vi "GetSlopeConductance3.vi"(8 "XYGraph Refnum":refnum<vi>, 10 "CapacitanceRecords":T2[](array[typedef]), 11 "Array in":dbl[][](array[numeric])) -> (1 "CleanedIV":cluster{dbl[], dbl[]}[](array[cluster]), 3 "InfoCluster":T1)   [LabVIEW 2020]
uses:
  CapacitanceRecord.ctl
  CapacitanceInfos.ctl
  <vilib>/Analysis/6fits.llb/Curve Fitting Criteria.ctl
  <vilib>/Analysis/NI_AALPro.lvlib
panel:
  out "error out":errorcluster
  out "XY Graph 2":cluster{dbl[], dbl[]}[](graph)
  out "XY Graph":cluster{dbl[], dbl[]}[](graph)
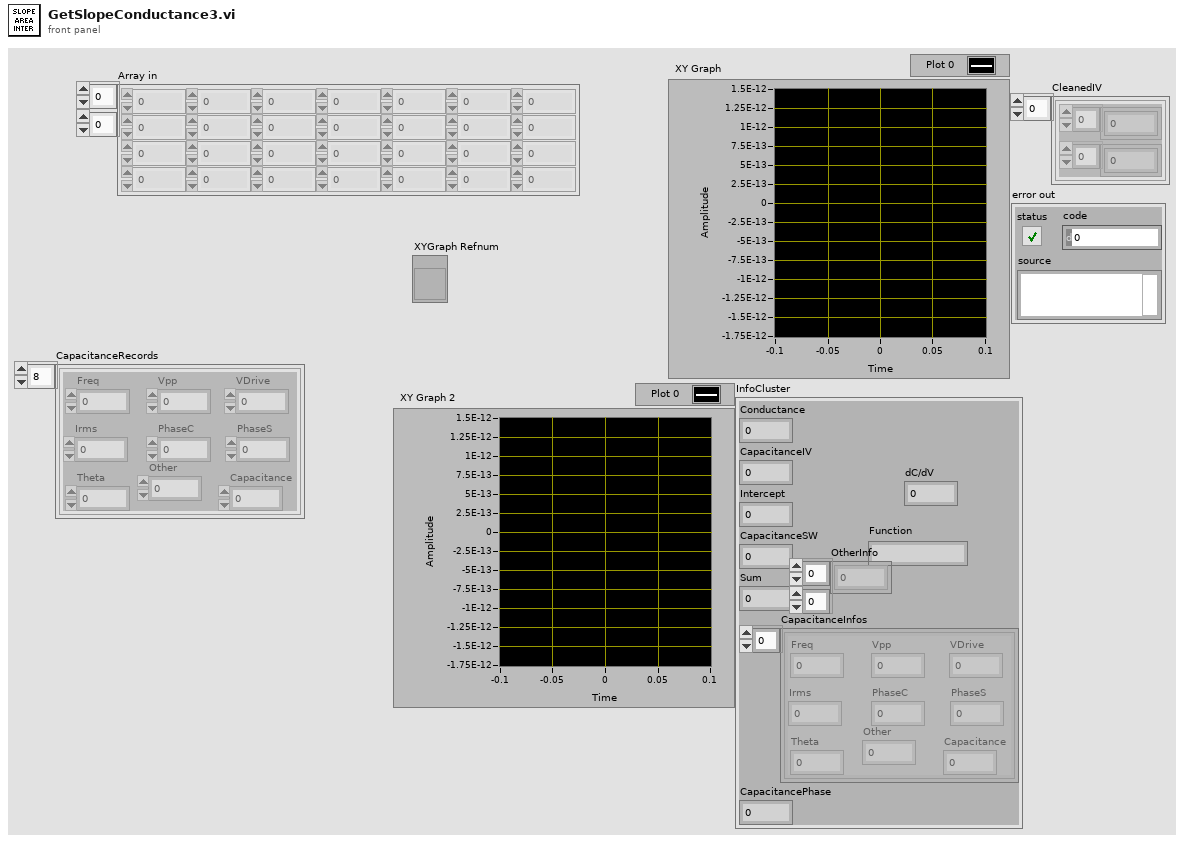
[diagram p1: front panel]
types:
  T1 = typedef "CapacitanceInfos.ctl" = cluster{"Conductance":dbl, "CapacitanceIV":dbl, "Intercept":dbl, "CapacitanceSW":dbl, "Sum":dbl, "CapacitanceInfos":T2[], "CapacitancePhase":dbl, "dC/dV":dbl, "Function":string, "OtherInfo":dbl[][]}
  T2 = typedef "CapacitanceRecord.ctl" = cluster{"Freq":dbl, "Vpp":dbl, "PhaseS":dbl, "Irms":dbl, "PhaseC":dbl, "Theta":dbl, "VDrive":dbl, "Capacitance":dbl, "Other":dbl}
  T3 = typedef "NI_AALPro.lvlib/Curve Fitting Criteria.ctl" = u16
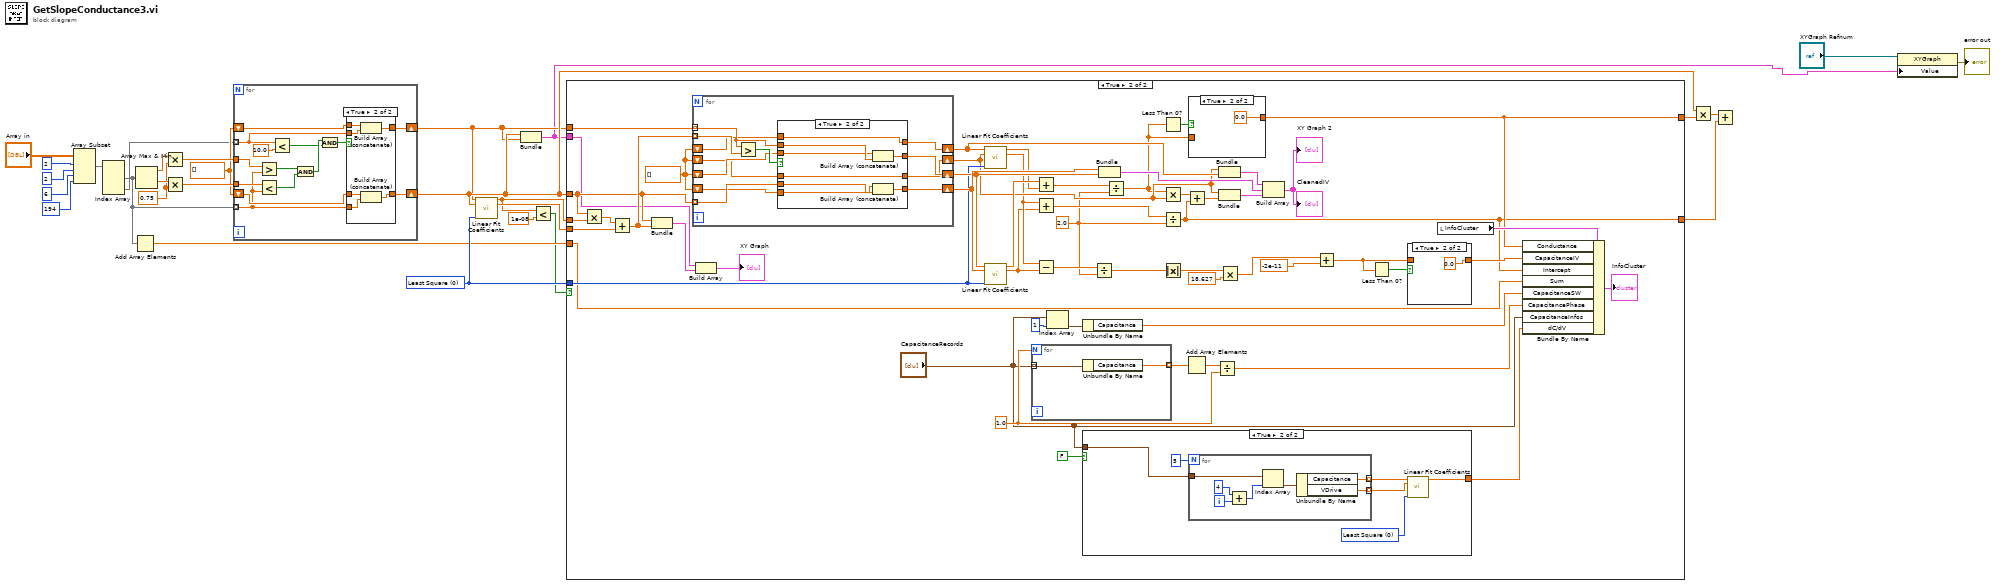
[diagram p0: block diagram]
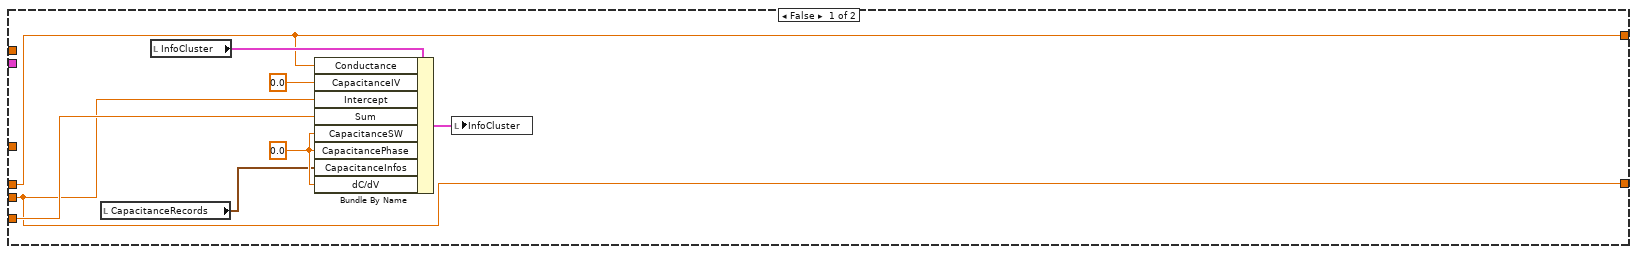
[diagram p2: hidden frame]
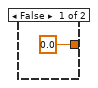
[diagram p3: hidden frame]
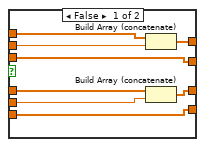
[diagram p6: hidden frame]
diagram:
  w17 = dbl[] []
  w16 = 0.75
  w12 = T3 0 items=["Least Square", "Least Absolute Residual", "Bisquare"] ("method")
  n1 = Array Subset(array="Array in", index (row)=2 ("index"), length (row)=2 ("length"), index (col)=6 ("index"), length (col)=194 ("length")) -> (w27:dbl[][])
  n2 = Index Array(array=w27) -> (element #1=w11:dbl[], element #2=w14:dbl[])  [unwired: 4 in]
  n3 = Add Array Elements(numeric array=w11) -> (sum=w10:dbl)
  n4 = Array Max & Min(array=w11) -> (max value=w21:dbl, min value=w20:dbl)  [unwired: 2 out]
  n5 = Multiply(x=w21, y=w16) -> (x*y=w19:dbl)
  n6 = Multiply(x=w20, y=w16) -> (x*y=w18:dbl)
  n7 = for {
    tunnel: w19 -> [w39]
    tunnel: w18 -> [w38]
    tunnel: w11 -> [w33] mode=indexing
    tunnel: w14 -> [w32] mode=indexing
    shift-right: [w35] -> w15
    shift-left: w17 -> [w37]
    shift-right: [w34] -> w13
    shift-left: w17 -> [w36]
    n8 = Greater?(x=w39, y=w33) -> (0:w42:bool)
    n9 = Less?(x=w38, y=w33) -> (x < y?=w41:bool)
    n10 = Less?(x=w32, y=10.0) -> (x < y?=w29:bool)
    n11 = And(x=w42, y=w41) -> (x .and. y?=w40:bool)
    n12 = And(x=w40, y=w29) -> (x .and. y?=w30:bool)
    n13 = case shown="True" w30 {
      tunnel: w37 -> [w44 w50]
      tunnel: w36 -> [w43 w49]
      tunnel: [w44 w48] -> w35
      tunnel: [w43 w47] -> w34
      tunnel: w33 -> [_ w46]
      tunnel: w32 -> [_ w45]
      frame False {
      }
      frame True {
        n14 = Build Array (concatenate)(w49, w45) -> (w47:dbl[])
        n15 = Build Array (concatenate)(w50, w46) -> (w48:dbl[])
      }
    }
  }
  n16 = call <vilib>:"Linear Fit Coefficients.vi"("Y"=w13, "X"=w15, "method"=w12) -> ("slope"=w8:dbl, "intercept"=w22:dbl)  [unwired: 10 in, 1 out]
  n17 = Bundle(w15, w13) -> (w3:cluster{dbl[], dbl[]})  [unwired: 1 in]
  n18 = Less?(x=w8, y=1e-08) -> (x < y?=w9:bool)
  n19 = case shown="True" w9 {
    tunnel: w8 -> [w52 w112]
    tunnel: w22 -> [w51 w110]
    tunnel: w15 -> [_ w62]
    tunnel: w13 -> [_ w102]
    tunnel: w12 -> [_ w98]
    tunnel: w10 -> [w56 w75]
    tunnel: [w52 w61] -> w6
    tunnel: [w51 w60] -> w5
    tunnel: w3 -> [_ w59]
    frame False {
      w54 = 0.0 ("CapacitanceSW")
      n20 = local read "CapacitanceRecords"() -> (w53:T2[])
      n21 = local read "InfoCluster"() -> (w58:T1)
      n22 = Bundle By Name(cluster=w58, "Conductance"=w52, "CapacitanceIV"=0.0, "Intercept"=w51, "Sum"=w56, "CapacitanceSW"=w54, "CapacitancePhase"=w54, "CapacitanceInfos"=w53, "dC/dV"=w54) -> (w57:T1)
      n23 = local write "InfoCluster"(w57) -> ()
    }
    frame True {
      w70 = 1.0 ("y")
      w86 = 2.0 ("y")
      w106 = dbl[] []
      n24 = Multiply(x=w62, y=w112) -> (x*y=w111:dbl[])
      n25 = Add(x=w111, y=w110) -> (x+y=w107:dbl[])
      n26 = Bundle(w62, w107) -> (w108:cluster{dbl[], dbl[]})  [unwired: 1 in]
      n27 = for {
        tunnel: w102 -> [w141] mode=indexing
        tunnel: w107 -> [w142] mode=indexing
        tunnel: w62 -> [w143] mode=indexing
        shift-right: [w139] -> w100
        shift-left: w106 -> [w137]
        shift-right: [w136] -> w91
        shift-left: w106 -> [w135]
        shift-right: [w140] -> w99
        shift-left: w106 -> [w138]
        shift-right: [w134] -> w101
        shift-left: w106 -> [w133]
        n28 = Greater?(x=w141, y=w142) -> (0:w144:bool)
        n29 = case shown="True" w144 {
          tunnel: w143 -> [w150 w159]
          tunnel: w141 -> [w146 w160]
          tunnel: [w151 w158] -> w139
          tunnel: [w152 w157] -> w140
          tunnel: w138 -> [w152 w156]
          tunnel: w137 -> [w151 w155]
          tunnel: [w149 w154] -> w136
          tunnel: w135 -> [w147 w154]
          tunnel: [w145 w153] -> w134
          tunnel: w133 -> [w148 w153]
          frame False {
            n30 = Build Array (concatenate)(w148, w146) -> (w145:dbl[])
            n31 = Build Array (concatenate)(w147, w150) -> (w149:dbl[])
          }
          frame True {
            n32 = Build Array (concatenate)(w156, w160) -> (w157:dbl[])
            n33 = Build Array (concatenate)(w155, w159) -> (w158:dbl[])
          }
        }
      }
      n34 = Build Array(w59, w108) -> (→"XY Graph":cluster{dbl[], dbl[]}[])
      n35 = call <vilib>:"Linear Fit Coefficients.vi"("Y"=w101, "X"=w91, "method"=w98) -> ("slope"=w96:dbl, "intercept"=w89:dbl)  [unwired: 10 in, 1 out]
      n36 = call <vilib>:"Linear Fit Coefficients.vi"("Y"=w99, "X"=w100, "method"=w98) -> ("slope"=w97:dbl, "intercept"=w88:dbl)  [unwired: 10 in, 1 out]
      n37 = for {
        N: w70 -> [_]
        tunnel: "CapacitanceRecords" -> [w130] mode=indexing
        tunnel: [w129] -> w73 mode=indexing
        n38 = Unbundle By Name(w130) -> ("Capacitance"=w129:dbl)
      }
      n39 = Add(x=w97, y=w96) -> (x+y=w95:dbl)
      n40 = Add(x=w89, y=w88) -> (x+y=w94:dbl)
      n41 = Subtract(x=w89, y=w88) -> (x-y=w87:dbl)
      n42 = Index Array(array="CapacitanceRecords", index=1) -> (element=w77:T2)
      n43 = Unbundle By Name(w77) -> ("Capacitance"=w74:dbl)
      n44 = case shown="True" FALSE {
        tunnel: "CapacitanceRecords" -> [_ w119]
        tunnel: [0.0 ("slope") w114] -> w66
        frame False {
        }
        frame True {
          w115 = T3 0 items=["Least Square", "Least Absolute Residual", "Bisquare"] ("method")
          n45 = for {
            N: 5 -> [_]
            tunnel: w119 -> [w126]
            tunnel: [w125] -> w116 mode=indexing
            tunnel: [w120] -> w117 mode=indexing
            i -> [w123]
            n46 = Add(x=4, y=w123) -> (x+y=w122:i32)
            n47 = Index Array(array=w126, index=w122) -> (element=w124:T2)
            n48 = Unbundle By Name(w124) -> ("Capacitance"=w125:dbl, "VDrive"=w120:dbl)
          }
          n49 = call <vilib>:"Linear Fit Coefficients.vi"("Y"=w116, "X"=w117, "method"=w115) -> ("slope"=w114:dbl)  [unwired: 10 in, 2 out]
        }
      }
      n50 = Divide(x=w87, y=w86) -> (x/y=w81:dbl)
      n51 = Bundle(w100, w99) -> (w104:cluster{dbl[], dbl[]})  [unwired: 1 in]
      n52 = Divide(x=w95, y=w86) -> (x/y=w64:dbl)
      n53 = Less Than 0?(x=w64) -> (x < 0?=w65:bool)
      n54 = Multiply(x=w64, y=w91) -> (x*y=w93:dbl[])
      n55 = Divide(x=w94, y=w86) -> (x/y=w60:dbl)
      n56 = Absolute Value(x=w81) -> (abs(x)=w85:dbl)
      n57 = Add(x=w93, y=w60) -> (x+y=w92:dbl[])
      n58 = Add Array Elements(numeric array=w73) -> (sum=w72:dbl)
      n59 = case shown="True" w65 {
        tunnel: [w127 0.0] -> w61
        tunnel: w64 -> [w127 _]
        frame False {
        }
        frame True {
        }
      }
      n60 = Divide(x=w72, y=w70) -> (x/y=w71:dbl)
      n61 = Bundle(w91, w101) -> (w103:cluster{dbl[], dbl[]})  [unwired: 1 in]
      n62 = Bundle(w91, w92) -> (w90:cluster{dbl[], dbl[]})  [unwired: 1 in]
      n63 = Multiply(x=w85, y=18.627) -> (x*y=w84:dbl)
      n64 = Build Array(w103, w104, w90) -> (→"XY Graph 2" →"CleanedIV":cluster{dbl[], dbl[]}[])
      n65 = Add(x=w84, y=-2e-11) -> (x+y=w79:dbl)
      n66 = Less Than 0?(x=w79) -> (x < 0?=w80:bool)
      n67 = case shown="True" w80 {
        tunnel: [w131 0.0] -> w76
        tunnel: w79 -> [w131 _]
        frame False {
        }
        frame True {
        }
      }
      n68 = local read "InfoCluster"() -> (w68:T1)
      n69 = Bundle By Name(cluster=w68, "Conductance"=w61, "CapacitanceIV"=w76, "Intercept"=w60, "Sum"=w75, "CapacitanceSW"=w74, "CapacitancePhase"=w71, "CapacitanceInfos"="CapacitanceRecords", "dC/dV"=w66) -> (→"InfoCluster":T1)
    }
  }
  n70 = Multiply(x=w15, y=w6) -> (x*y=w4:dbl[])
  n71 = Add(x=w4, y=w5) -> ()  [unwired: 1 out]
  n72 = property class="XYGraph"(reference="XYGraph Refnum", "Value"=w3) -> (error out=→"error out":errorcluster)  [unwired: 1 in, 1 out]
